vi "buy.vi"(8 "error in (no error)":errorcluster, 11 "Stock in":refnum<class "Stock.lvclass">) -> (0 "error out":errorcluster, 3 "Stock out":refnum<class "Stock.lvclass">)   [LabVIEW 2017, in "Stock.lvclass"]
uses:
  Stock.lvclass
  Stock.lvclass/Stock.ctl
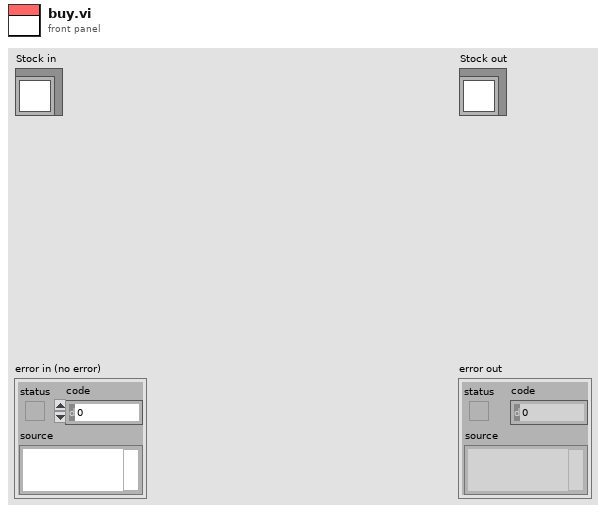
[diagram p1: front panel]
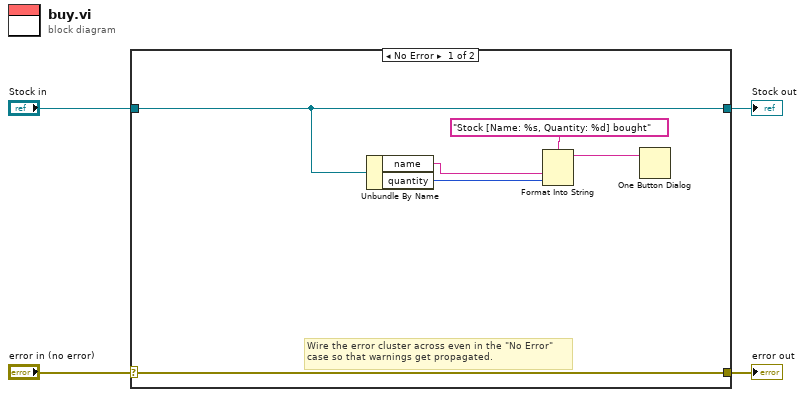
[diagram p0: block diagram]
diagram:
  n1 = case shown="No Error" "error in (no error)" {
    selector: "error in (no error)" -> [w10 w12]
    tunnel: [w10 w12] -> w3
    tunnel: [w9 w11] -> w1
    tunnel: "Stock in" -> [w9 w11]
    frame No Error {
      # "Wire the error cluster across even in the \"No Error\"\ncase so that warnings get propagated."
      n2 = Unbundle By Name(w9) -> ("name"=w7:string, "quantity"=w6:u8)
      n3 = Format Into String(format string="Stock [Name: %s, Quantity: %d] bought", w7, w6) -> (resulting string=w5:string)  [unwired: 2 in, 1 out]
      n4 = One Button Dialog(message=w5) -> ()  [unwired: 1 in, 1 out]
    }
    frame Error {
    }
  }
  "error out" <- w3
  "Stock out" <- w1
